vi "send frame.vi"(8 "error in (no error)":errorcluster, 10 "Voltage array":u16[](array[numeric]), 11 "BMC in":refnum<class "BMC.lvclass">) -> (0 "error out":errorcluster, 3 "BMC out":refnum<class "BMC.lvclass">)   [LabVIEW 2012, in "BMC.lvclass"]
uses:
  BMC.lvclass
  BMC.lvclass/BMC.ctl
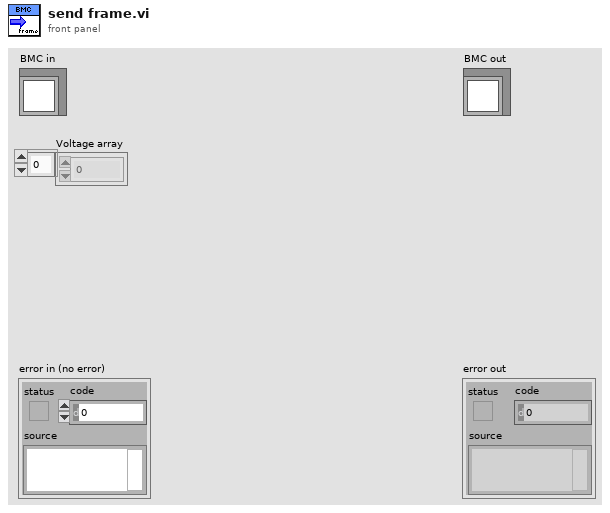
[diagram p1: front panel]
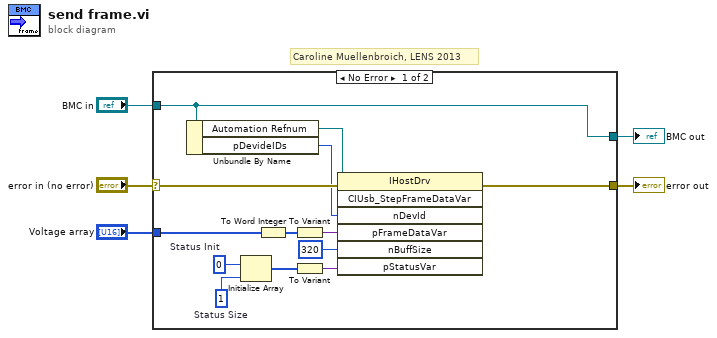
[diagram p0: block diagram]
diagram:
  # "Caroline Muellenbroich, LENS 2013"
  n1 = case shown="No Error" "error in (no error)" {
    selector: "error in (no error)" -> [w15 w20]
    tunnel: [w7 w20] -> w4
    tunnel: [w6 w19] -> w2
    tunnel: "BMC in" -> [w6 w19]
    tunnel: "Voltage array" -> [w12 _]
    frame No Error {
      w10 = 1  # Status Size
      w11 = 0  # Status Init
      n2 = Unbundle By Name(w6) -> ("Automation Refnum"=w13:refnum<k7>, "pDevideIDs"=w14:i32)
      n3 = Initialize Array(w11, w10) -> (w9:i32[])
      n4 = To Word Integer(number=w12) -> (16bit integer=w8:i16[])
      n5 = To Variant(anything=w8) -> (Variant=w16:variant)
      n6 = To Variant(anything=w9) -> (Variant=w17:variant)
      n7 = invoke class="IHostDrv" method="CIUsb_StepFrameDataVar"(reference=w13, error in=w15, "nDevId"=w14, "pFrameDataVar"=w16, "nBuffSize"=320, "pStatusVar"=w17) -> (error out=w7:errorcluster)  [unwired: 1 in, 6 out]
    }
    frame Error {
    }
  }
  "error out" <- w4
  "BMC out" <- w2
